vi "Passmark_Setting_Save.vi"(7 "Table_Data 2":refnum<vi>, 8 "error in (no error)":errorcluster caption="错误输入（无错误）", 9 "GRR_Title_Setting_path":path=path "D:/Desktop/?????/Title_RecipeEVT3_GRR.csv", 10 "Title_Setting_path":path=path "D:/Desktop/?????/Title_RecipeEVT3.csv", 11 "Flow_Setting_path":path=path "D:/Desktop/?????/EOL_Passmark_Setting_RecipeEVT3.csv") -> (0 "error out":errorcluster caption="错误输出")   [LabVIEW 2017]
uses:
  <vilib>/Utility/file.llb/Read Delimited Spreadsheet (string).vi
  <vilib>/Utility/file.llb/Write Delimited Spreadsheet (string).vi
panel:
  out "GRR_Title_Setting_path 2":path
  out "Title_Setting_path 2":path
  out "Flow_Setting_path 2":path
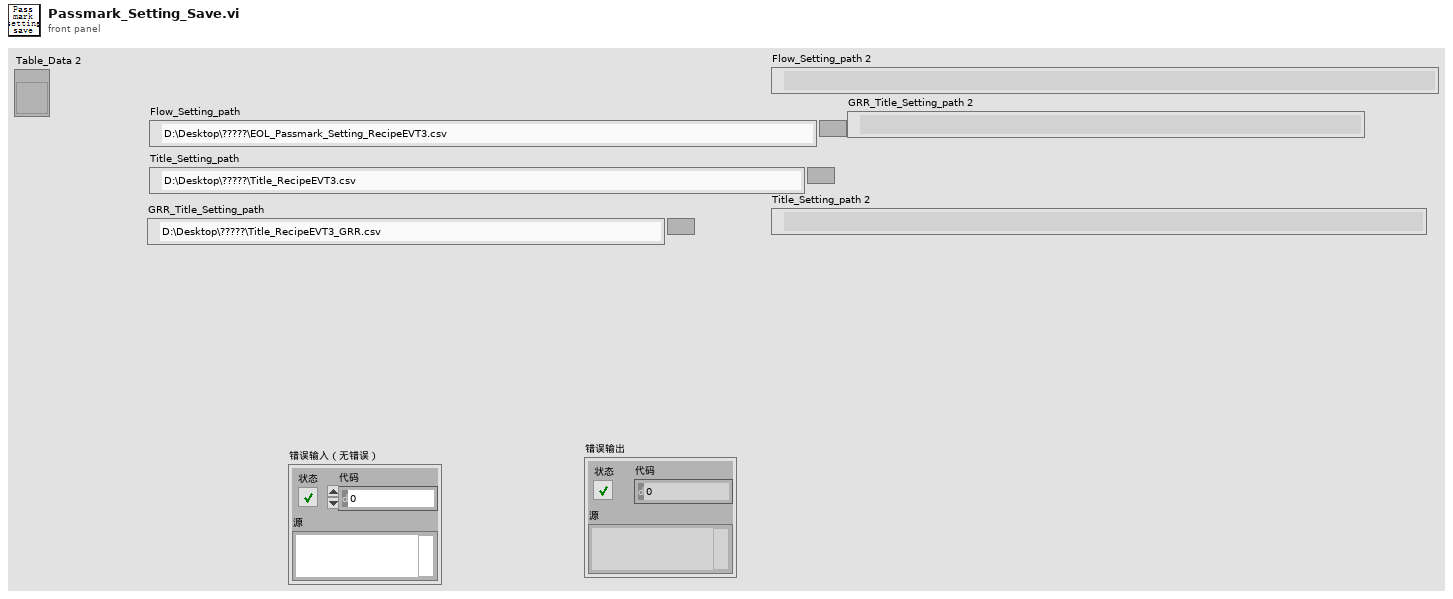
[diagram p1: front panel]
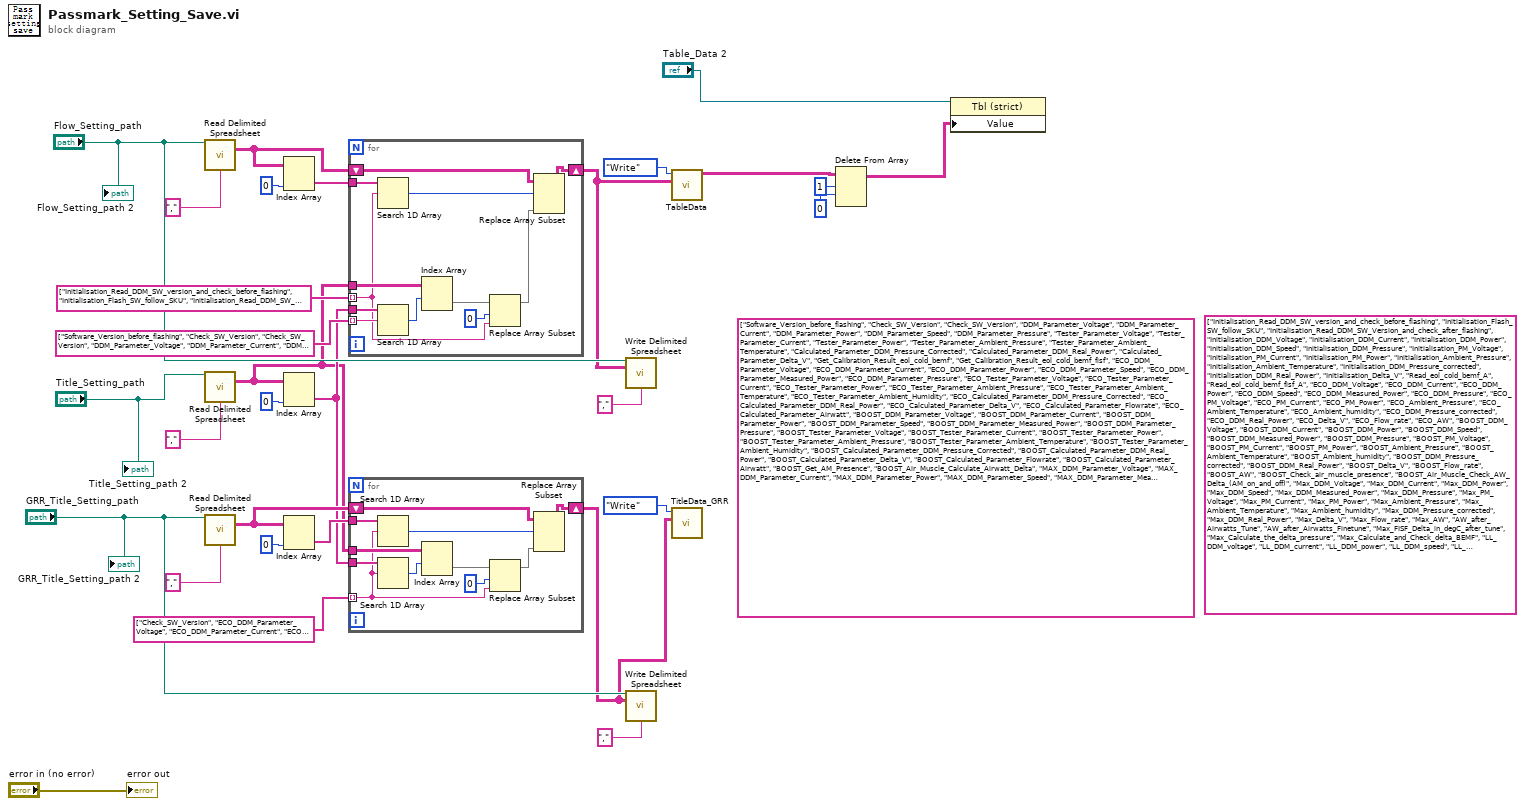
[diagram p0: block diagram]
diagram:
  (unwired) string[] ["Initialisation_Read_DDM_SW_version_and_check_before_flashing", "Initialisation_Flash_SW_follow_SKU", "Initialisation_Read_DDM_SW_Version_and_check_after_flashing", "Initialisation_DDM_Voltage", "Initialisation_DDM_Current", "Initialisation_DDM_Power", "Initialisation_DDM_Speed", "Initialisation_DDM_Pressure", "Initialisation_PM_Voltage", "Initialisation_PM_Current", "Initialisation_PM_Power", "Initialisation_Ambient_Pressure", "Initialisation_Ambient_Temperature", "Initialisation_DDM_Pressure_corrected", "Initialisation_DDM_Real_Power", "Initialisation_Delta_V", "Read_eol_cold_bemf_A", "Read_eol_cold_bemf_fisf_A", "ECO_DDM_Voltage", "ECO_DDM_Current", "ECO_DDM_Power", "ECO_DDM_Speed", "ECO_DDM_Measured_Power", "ECO_DDM_Pressure", "ECO_PM_Voltage", "ECO_PM_Current", "ECO_PM_Power", "ECO_Ambient_Pressure", "ECO_Ambient_Temperature", "ECO_Ambient_humidity", "ECO_DDM_Pressure_corrected", "ECO_DDM_Real_Power", "ECO_Delta_V", "ECO_Flow_rate", "ECO_AW", "BOOST_DDM_Voltage", "BOOST_DDM_Current", "BOOST_DDM_Power", "BOOST_DDM_Speed", "BOOST_DDM_Measured_Power", "BOOST_DDM_Pressure", "BOOST_PM_Voltage", "BOOST_PM_Current", "BOOST_PM_Power", "BOOST_Ambient_Pressure", "BOOST_Ambient_Temperature", "BOOST_Ambient_humidity", "BOOST_DDM_Pressure_corrected", "BOOST_DDM_Real_Power", "BOOST_Delta_V", "BOOST_Flow_rate", "BOOST_AW", "BOOST_Check_air_muscle_presence", "BOOST_Air_Muscle_Check_AW_Delta_(AM_on_and_off)", "Max_DDM_Voltage", "Max_DDM_Current", "Max_DDM_Power", "Max_DDM_Speed", "Max_DDM_Measured_Power", "Max_DDM_Pressure", "Max_PM_Voltage", "Max_PM_Current", "Max_PM_Power", "Max_Ambient_Pressure", "Max_Ambient_Temperature", "Max_Ambient_humidity", "Max_DDM_Pressure_corrected", "Max_DDM_Real_Power", "Max_Delta_V", "Max_Flow_rate", "Max_AW", "AW_after_Airwatts_Tune", "AW_after_Airwatts_Finetune", "Max_FISF_Delta_in_degC_after_tune", "Max_Calculate_the_delta_pressure", "Max_Calculate_and_Check_delta_BEMF", "LL_DDM_voltage", "LL_DDM_current", "LL_DDM_power", "LL_DDM_speed", "LL_DDM_measured_power", "LL_DDM_pressure", "LL_Tester_Voltage", "LL_Tester_Current", "LL_Tester_Power", "LL_DDM_Real_Power", "Calibrate_task_detect-LL(A)", "HL_DDM_voltage", "HL_DDM_current", "HL_DDM_power", "HL_DDM_speed", "HL_DDM_measured_power", "HL_DDM_pressure", "HL_Tester_Voltage", "HL_Tester_Current", "HL_Tester_Power", "HL_DDM_Real_Power", "Calibrate_task_detect-HL(B)", "LH_DDM_voltage", "LH_DDM_current", "LH_DDM_power", "LH_DDM_speed", "LH_DDM_measured_power", "LH_DDM_pressure", "LH_Tester_Voltage", "LH_Tester_Current", "LH_Tester_Power", "LH_DDM_Real_Power", "Calibrate_task_detect-LH(C)", "HH_DDM_voltage", "HH_DDM_current", "HH_DDM_power", "HH_DDM_speed", "HH_DDM_measured_power", "HH_DDM_pressure", "HH_Tester_Voltage", "HH_Tester_Current", "HH_Tester_Power", "HH_DDM_Real_Power", "Calibrate_task_detect-HH(D)", "Inlet_Blockage_Calibration_DDM_voltage", "Inlet_Blockage_Calibration_DDM_current", "Inlet_Blockage_Calibration_DDM_power", "Inlet_Blockage_Calibration_DDM_speed", "Inlet_Blockage_Calibration_DDM_measured_power", "Inlet_Blockage_Calibration_pressure", "Inlet_Blockage_Calibration_Tester_Voltage", "Inlet_Blockage_Calibration_Tester_Current", "Inlet_Blockage_Calibration_Tester_Power", "Inlet_Blockage_Calibration_DDM_Real_Power", "HH_Get_inlet_blockage_calibration(E)"] ("子数组 3")
  (unwired) string[] ["Software_Version_before_flashing", "Check_SW_Version", "Check_SW_Version", "DDM_Parameter_Voltage", "DDM_Parameter_Current", "DDM_Parameter_Power", "DDM_Parameter_Speed", "DDM_Parameter_Pressure", "Tester_Parameter_Voltage", "Tester_Parameter_Current", "Tester_Parameter_Power", "Tester_Parameter_Ambient_Pressure", "Tester_Parameter_Ambient_Temperature", "Calculated_Parameter_DDM_Pressure_Corrected", "Calculated_Parameter_DDM_Real_Power", "Calculated_Parameter_Delta_V", "Get_Calibration_Result_eol_cold_bemf", "Get_Calibration_Result_eol_cold_bemf_fisf", "ECO_DDM_Parameter_Voltage", "ECO_DDM_Parameter_Current", "ECO_DDM_Parameter_Power", "ECO_DDM_Parameter_Speed", "ECO_DDM_Parameter_Measured_Power", "ECO_DDM_Parameter_Pressure", "ECO_Tester_Parameter_Voltage", "ECO_Tester_Parameter_Current", "ECO_Tester_Parameter_Power", "ECO_Tester_Parameter_Ambient_Pressure", "ECO_Tester_Parameter_Ambient_Temperature", "ECO_Tester_Parameter_Ambient_Humidity", "ECO_Calculated_Parameter_DDM_Pressure_Corrected", "ECO_Calculated_Parameter_DDM_Real_Power", "ECO_Calculated_Parameter_Delta_V", "ECO_Calculated_Parameter_Flowrate", "ECO_Calculated_Parameter_Airwatt", "BOOST_DDM_Parameter_Voltage", "BOOST_DDM_Parameter_Current", "BOOST_DDM_Parameter_Power", "BOOST_DDM_Parameter_Speed", "BOOST_DDM_Parameter_Measured_Power", "BOOST_DDM_Parameter_Pressure", "BOOST_Tester_Parameter_Voltage", "BOOST_Tester_Parameter_Current", "BOOST_Tester_Parameter_Power", "BOOST_Tester_Parameter_Ambient_Pressure", "BOOST_Tester_Parameter_Ambient_Temperature", "BOOST_Tester_Parameter_Ambient_Humidity", "BOOST_Calculated_Parameter_DDM_Pressure_Corrected", "BOOST_Calculated_Parameter_DDM_Real_Power", "BOOST_Calculated_Parameter_Delta_V", "BOOST_Calculated_Parameter_Flowrate", "BOOST_Calculated_Parameter_Airwatt", "BOOST_Get_AM_Presence", "BOOST_Air_Muscle_Calculate_Airwatt_Delta", "MAX_DDM_Parameter_Voltage", "MAX_DDM_Parameter_Current", "MAX_DDM_Parameter_Power", "MAX_DDM_Parameter_Speed", "MAX_DDM_Parameter_Measured_Power", "MAX_DDM_Parameter_Pressure", "MAX_Tester_Parameter_Voltage", "MAX_Tester_Parameter_Current", "MAX_Tester_Parameter_Power", "MAX_Tester_Parameter_Ambient_Pressure", "MAX_Tester_Parameter_Ambient_Temperature", "MAX_Tester_Parameter_Ambient_Humidity", "MAX_Calculated_Parameter_DDM_Pressure_Corrected", "MAX_Calculated_Parameter_DDM_Real_Power", "MAX_Calculated_Parameter_Delta_V", "MAX_Calculated_Parameter_Flowrate", "MAX_Calculated_Parameter_Airwatt", "MAX_tune_Calculated_Parameter_Airwatt", "MAX_finetune_Calculated_Parameter_Airwatt", "Delta_Tmag_FISF", "Calculate_delta_Pressure", "Calculate_Check_Delta_BEMF", "LL_DDM_Parameter_Voltage", "LL_DDM_Parameter_Current", "LL_DDM_Parameter_Power", "LL_DDM_Parameter_Speed", "LL_DDM_Parameter_Measured_Power", "LL_DDM_Parameter_Pressure", "LL_Tester_Parameter_Voltage", "LL_Tester_Parameter_Current", "LL_Tester_Parameter_Power", "LL_DDM_Real_Power", "LL_Calibrate_Task_Detect_LL", "HL_DDM_Parameter_Voltage", "HL_DDM_Parameter_Current", "HL_DDM_Parameter_Power", "HL_DDM_Parameter_Speed", "HL_DDM_Parameter_Measured_Power", "HL_DDM_Parameter_Pressure", "HL_Tester_Parameter_Voltage", "HL_Tester_Parameter_Current", "HL_Tester_Parameter_Power", "HL_DDM_Real_Power", "HL_Calibrate_Task_Detect_HL", "LH_DDM_Parameter_Voltage", "LH_DDM_Parameter_Current", "LH_DDM_Parameter_Power", "LH_DDM_Parameter_Speed", "LH_DDM_Parameter_Measured_Power", "LH_DDM_Parameter_Pressure", "LH_Tester_Parameter_Voltage", "LH_Tester_Parameter_Current", "LH_Tester_Parameter_Power", "LH_DDM_Real_Power", "LH_Calibrate_Task_Detect_LH", "HH_DDM_Parameter_Voltage", "HH_DDM_Parameter_Current", "HH_DDM_Parameter_Power", "HH_DDM_Parameter_Speed", "HH_DDM_Parameter_Measured_Power", "HH_DDM_Parameter_Pressure", "HH_Tester_Parameter_Voltage", "HH_Tester_Parameter_Current", "HH_Tester_Parameter_Power", "HH_DDM_Real_Power", "HH_Calibrate_Task_Detect_HH", "Inlet_Blockage_Calibration_DDM_Parameter_Voltage", "Inlet_Blockage_Calibration_DDM_Parameter_Current", "Inlet_Blockage_Calibration_DDM_Parameter_Power", "Inlet_Blockage_Calibration_DDM_Parameter_Speed", "Inlet_Blockage_Calibration_DDM_Parameter_Measured_Power", "Inlet_Blockage_Calibration_DDM_Parameter_Pressure", "Inlet_Blockage_Calibration_Tester_Parameter_Voltage", "Inlet_Blockage_Calibration_Tester_Parameter_Current", "Inlet_Blockage_Calibration_Tester_Parameter_Power", "Inlet_Blockage_Calibration_DDM_Real_Power", "Calibration_Inlet_Blockage"] ("子数组 3")
  n1 = call-poly <vilib>:"Read Delimited Spreadsheet.vi"("file path (dialog if empty)"="Flow_Setting_path", "delimiter (\\t)"="," ("delimiter (\\t)")) -> ("all rows"=w25:string[][])  [unwired: 8 in, 5 out]
  n2 = call-poly <vilib>:"Read Delimited Spreadsheet.vi"("file path (dialog if empty)"="Title_Setting_path", "delimiter (\\t)"="," ("delimiter (\\t)")) -> ("all rows"=w11:string[][])  [unwired: 8 in, 5 out]
  n3 = call-poly <vilib>:"Read Delimited Spreadsheet.vi"("file path (dialog if empty)"="GRR_Title_Setting_path", "delimiter (\\t)"="," ("delimiter (\\t)")) -> ("all rows"=w18:string[][])  [unwired: 8 in, 5 out]
  n4 = Index Array(array=w25, index (col)=0 ("禁用的索引 (列)")) -> (element=w22:string[])  [unwired: 1 in]
  n5 = Index Array(array=w11, index (col)=0 ("禁用的索引 (列)")) -> (element=w12:string[])  [unwired: 1 in]
  n6 = Index Array(array=w18, index (col)=0 ("禁用的索引 (列)")) -> (element=w17:string[])  [unwired: 1 in]
  n7 = for {
    tunnel: string[] ["Initialisation_Read_DDM_SW_version_and_check_before_flashing", "Initialisation_Flash_SW_follow_SKU", "Initialisation_Read_DDM_SW_Version_and_check_after_flashing", "Initialisation_DDM_Voltage", "Initialisation_DDM_Current", "Initialisation_DDM_Power", "Initialisation_DDM_Speed", "Initialisation_DDM_Pressure", "Initialisation_PM_Voltage", "Initialisation_PM_Current", "Initialisation_PM_Power", "Initialisation_Ambient_Pressure", "Initialisation_Ambient_Temperature", "Initialisation_DDM_Pressure_corrected", "Initialisation_DDM_Real_Power", "Initialisation_Delta_V", "Read_eol_cold_bemf_A", "Read_eol_cold_bemf_fisf_A", "ECO_DDM_Voltage", "ECO_DDM_Current", "ECO_DDM_Power", "ECO_DDM_Speed", "ECO_DDM_Measured_Power", "ECO_DDM_Pressure", "ECO_PM_Voltage", "ECO_PM_Current", "ECO_PM_Power", "ECO_Ambient_Pressure", "ECO_Ambient_Temperature", "ECO_Ambient_humidity", "ECO_DDM_Pressure_corrected", "ECO_DDM_Real_Power", "ECO_Delta_V", "ECO_Flow_rate", "ECO_AW", "BOOST_DDM_Voltage", "BOOST_DDM_Current", "BOOST_DDM_Power", "BOOST_DDM_Speed", "BOOST_DDM_Measured_Power", "BOOST_DDM_Pressure", "BOOST_PM_Voltage", "BOOST_PM_Current", "BOOST_PM_Power", "BOOST_Ambient_Pressure", "BOOST_Ambient_Temperature", "BOOST_Ambient_humidity", "BOOST_DDM_Pressure_corrected", "BOOST_DDM_Real_Power", "BOOST_Delta_V", "BOOST_Flow_rate", "BOOST_AW", "BOOST_Check_air_muscle_presence", "BOOST_Air_Muscle_Check_AW_Delta_(AM_on_and_off)", "Max_DDM_Voltage", "Max_DDM_Current", "Max_DDM_Power", "Max_DDM_Speed", "Max_DDM_Measured_Power", "Max_DDM_Pressure", "Max_PM_Voltage", "Max_PM_Current", "Max_PM_Power", "Max_Ambient_Pressure", "Max_Ambient_Temperature", "Max_Ambient_humidity", "Max_DDM_Pressure_corrected", "Max_DDM_Real_Power", "Max_Delta_V", "Max_Flow_rate", "Max_AW", "AW_after_Airwatts_Tune", "AW_after_Airwatts_Finetune", "Max_FISF_Delta_in_degC_after_tune", "Max_Calculate_the_delta_pressure", "Max_Calculate_and_Check_delta_BEMF", "LL_DDM_voltage", "LL_DDM_current", "LL_DDM_power", "LL_DDM_speed", "LL_DDM_measured_power", "LL_DDM_pressure", "LL_Tester_Voltage", "LL_Tester_Current", "LL_Tester_Power", "LL_DDM_Real_Power", "Calibrate_task_detect-LL(A)", "HL_DDM_voltage", "HL_DDM_current", "HL_DDM_power", "HL_DDM_speed", "HL_DDM_measured_power", "HL_DDM_pressure", "HL_Tester_Voltage", "HL_Tester_Current", "HL_Tester_Power", "HL_DDM_Real_Power", "Calibrate_task_detect-HL(B)", "LH_DDM_voltage", "LH_DDM_current", "LH_DDM_power", "LH_DDM_speed", "LH_DDM_measured_power", "LH_DDM_pressure", "LH_Tester_Voltage", "LH_Tester_Current", "LH_Tester_Power", "LH_DDM_Real_Power", "Calibrate_task_detect-LH(C)", "HH_DDM_voltage", "HH_DDM_current", "HH_DDM_power", "HH_DDM_speed", "HH_DDM_measured_power", "HH_DDM_pressure", "HH_Tester_Voltage", "HH_Tester_Current", "HH_Tester_Power", "HH_DDM_Real_Power", "Calibrate_task_detect-HH(D)", "Inlet_Blockage_Calibration_DDM_voltage", "Inlet_Blockage_Calibration_DDM_current", "Inlet_Blockage_Calibration_DDM_power", "Inlet_Blockage_Calibration_DDM_speed", "Inlet_Blockage_Calibration_DDM_measured_power", "Inlet_Blockage_Calibration_pressure", "Inlet_Blockage_Calibration_Tester_Voltage", "Inlet_Blockage_Calibration_Tester_Current", "Inlet_Blockage_Calibration_Tester_Power", "Inlet_Blockage_Calibration_DDM_Real_Power", "HH_Get_inlet_blockage_calibration(E)"] ("子数组 3") -> [w33] mode=indexing
    tunnel: string[] ["Software_Version_before_flashing", "Check_SW_Version", "Check_SW_Version", "DDM_Parameter_Voltage", "DDM_Parameter_Current", "DDM_Parameter_Power", "DDM_Parameter_Speed", "DDM_Parameter_Pressure", "Tester_Parameter_Voltage", "Tester_Parameter_Current", "Tester_Parameter_Power", "Tester_Parameter_Ambient_Pressure", "Tester_Parameter_Ambient_Temperature", "Calculated_Parameter_DDM_Pressure_Corrected", "Calculated_Parameter_DDM_Real_Power", "Calculated_Parameter_Delta_V", "Get_Calibration_Result_eol_cold_bemf", "Get_Calibration_Result_eol_cold_bemf_fisf", "ECO_DDM_Parameter_Voltage", "ECO_DDM_Parameter_Current", "ECO_DDM_Parameter_Power", "ECO_DDM_Parameter_Speed", "ECO_DDM_Parameter_Measured_Power", "ECO_DDM_Parameter_Pressure", "ECO_Tester_Parameter_Voltage", "ECO_Tester_Parameter_Current", "ECO_Tester_Parameter_Power", "ECO_Tester_Parameter_Ambient_Pressure", "ECO_Tester_Parameter_Ambient_Temperature", "ECO_Tester_Parameter_Ambient_Humidity", "ECO_Calculated_Parameter_DDM_Pressure_Corrected", "ECO_Calculated_Parameter_DDM_Real_Power", "ECO_Calculated_Parameter_Delta_V", "ECO_Calculated_Parameter_Flowrate", "ECO_Calculated_Parameter_Airwatt", "BOOST_DDM_Parameter_Voltage", "BOOST_DDM_Parameter_Current", "BOOST_DDM_Parameter_Power", "BOOST_DDM_Parameter_Speed", "BOOST_DDM_Parameter_Measured_Power", "BOOST_DDM_Parameter_Pressure", "BOOST_Tester_Parameter_Voltage", "BOOST_Tester_Parameter_Current", "BOOST_Tester_Parameter_Power", "BOOST_Tester_Parameter_Ambient_Pressure", "BOOST_Tester_Parameter_Ambient_Temperature", "BOOST_Tester_Parameter_Ambient_Humidity", "BOOST_Calculated_Parameter_DDM_Pressure_Corrected", "BOOST_Calculated_Parameter_DDM_Real_Power", "BOOST_Calculated_Parameter_Delta_V", "BOOST_Calculated_Parameter_Flowrate", "BOOST_Calculated_Parameter_Airwatt", "BOOST_Get_AM_Presence", "BOOST_Air_Muscle_Calculate_Airwatt_Delta", "MAX_DDM_Parameter_Voltage", "MAX_DDM_Parameter_Current", "MAX_DDM_Parameter_Power", "MAX_DDM_Parameter_Speed", "MAX_DDM_Parameter_Measured_Power", "MAX_DDM_Parameter_Pressure", "MAX_Tester_Parameter_Voltage", "MAX_Tester_Parameter_Current", "MAX_Tester_Parameter_Power", "MAX_Tester_Parameter_Ambient_Pressure", "MAX_Tester_Parameter_Ambient_Temperature", "MAX_Tester_Parameter_Ambient_Humidity", "MAX_Calculated_Parameter_DDM_Pressure_Corrected", "MAX_Calculated_Parameter_DDM_Real_Power", "MAX_Calculated_Parameter_Delta_V", "MAX_Calculated_Parameter_Flowrate", "MAX_Calculated_Parameter_Airwatt", "MAX_tune_Calculated_Parameter_Airwatt", "MAX_finetune_Calculated_Parameter_Airwatt", "Delta_Tmag_FISF", "Calculate_delta_Pressure", "Calculate_Check_Delta_BEMF", "LL_DDM_Parameter_Voltage", "LL_DDM_Parameter_Current", "LL_DDM_Parameter_Power", "LL_DDM_Parameter_Speed", "LL_DDM_Parameter_Measured_Power", "LL_DDM_Parameter_Pressure", "LL_Tester_Parameter_Voltage", "LL_Tester_Parameter_Current", "LL_Tester_Parameter_Power", "LL_DDM_Real_Power", "LL_Calibrate_Task_Detect_LL", "HL_DDM_Parameter_Voltage", "HL_DDM_Parameter_Current", "HL_DDM_Parameter_Power", "HL_DDM_Parameter_Speed", "HL_DDM_Parameter_Measured_Power", "HL_DDM_Parameter_Pressure", "HL_Tester_Parameter_Voltage", "HL_Tester_Parameter_Current", "HL_Tester_Parameter_Power", "HL_DDM_Real_Power", "HL_Calibrate_Task_Detect_HL", "LH_DDM_Parameter_Voltage", "LH_DDM_Parameter_Current", "LH_DDM_Parameter_Power", "LH_DDM_Parameter_Speed", "LH_DDM_Parameter_Measured_Power", "LH_DDM_Parameter_Pressure", "LH_Tester_Parameter_Voltage", "LH_Tester_Parameter_Current", "LH_Tester_Parameter_Power", "LH_DDM_Real_Power", "LH_Calibrate_Task_Detect_LH", "HH_DDM_Parameter_Voltage", "HH_DDM_Parameter_Current", "HH_DDM_Parameter_Power", "HH_DDM_Parameter_Speed", "HH_DDM_Parameter_Measured_Power", "HH_DDM_Parameter_Pressure", "HH_Tester_Parameter_Voltage", "HH_Tester_Parameter_Current", "HH_Tester_Parameter_Power", "HH_DDM_Real_Power", "HH_Calibrate_Task_Detect_HH", "Inlet_Blockage_Calibration_DDM_Parameter_Voltage", "Inlet_Blockage_Calibration_DDM_Parameter_Current", "Inlet_Blockage_Calibration_DDM_Parameter_Power", "Inlet_Blockage_Calibration_DDM_Parameter_Speed", "Inlet_Blockage_Calibration_DDM_Parameter_Measured_Power", "Inlet_Blockage_Calibration_DDM_Parameter_Pressure", "Inlet_Blockage_Calibration_Tester_Parameter_Voltage", "Inlet_Blockage_Calibration_Tester_Parameter_Current", "Inlet_Blockage_Calibration_Tester_Parameter_Power", "Inlet_Blockage_Calibration_DDM_Real_Power", "Calibration_Inlet_Blockage"] ("子数组 3") -> [w41] mode=indexing
    tunnel: w11 -> [w39]
    tunnel: w12 -> [w42]
    tunnel: w22 -> [w40]
    shift-right: [w37] -> w8
    shift-left: w25 -> [w36]
    n8 = Search 1D Array(1D array=w40, element=w33) -> (index of element=w35:i32)  [unwired: 1 in]
    n9 = Search 1D Array(1D array=w42, element=w41) -> (index of element=w38:i32)  [unwired: 1 in]
    n10 = Index Array(array=w39, index (row)=w38) -> (element=w34:string[])  [unwired: 1 in]
    n11 = Replace Array Subset(array=w34, new element=w33, index=0 ("索引")) -> (w31:string[])
    n12 = Replace Array Subset ("替换数组子集")(array=w36, new element=w31, index (row)=w35) -> (w37:string[][])  [unwired: 1 in]
  }
  n13 = for {
    tunnel: string[] ["Check_SW_Version", "ECO_DDM_Parameter_Voltage", "ECO_DDM_Parameter_Current", "ECO_DDM_Parameter_Power", "ECO_DDM_Parameter_Measured_Power", "ECO_DDM_Parameter_Speed", "ECO_DDM_Parameter_Pressure", "ECO_Tester_Parameter_Voltage", "ECO_Tester_Parameter_Current", "ECO_Tester_Parameter_Power", "ECO_Tester_Parameter_Ambient_Pressure", "ECO_Tester_Parameter_Ambient_Temperature", "ECO_Tester_Parameter_Ambient_Humidity", "ECO_Calculated_Parameter_DDM_Pressure_Corrected", "ECO_Calculated_Parameter_DDM_Real_Power", "ECO_Calculated_Parameter_Delta_V", "ECO_Calculated_Parameter_Flowrate", "ECO_Calculated_Parameter_Airwatt", "BOOST_DDM_Parameter_Voltage", "BOOST_DDM_Parameter_Current", "BOOST_DDM_Parameter_Power", "BOOST_DDM_Parameter_Measured_Power", "BOOST_DDM_Parameter_Speed", "BOOST_DDM_Parameter_Pressure", "BOOST_Tester_Parameter_Voltage", "BOOST_Tester_Parameter_Current", "BOOST_Tester_Parameter_Power", "BOOST_Tester_Parameter_Ambient_Pressure", "BOOST_Tester_Parameter_Ambient_Temperature", "BOOST_Tester_Parameter_Ambient_Humidity", "BOOST_Calculated_Parameter_DDM_Pressure_Corrected", "BOOST_Calculated_Parameter_DDM_Real_Power", "BOOST_Calculated_Parameter_Delta_V", "BOOST_Calculated_Parameter_Flowrate", "BOOST_Calculated_Parameter_Airwatt", "MAX_DDM_Parameter_Voltage", "MAX_DDM_Parameter_Current", "MAX_DDM_Parameter_Power", "MAX_DDM_Parameter_Measured_Power", "MAX_DDM_Parameter_Speed", "MAX_DDM_Parameter_Pressure", "MAX_Tester_Parameter_Voltage", "MAX_Tester_Parameter_Current", "MAX_Tester_Parameter_Power", "MAX_Tester_Parameter_Ambient_Pressure", "MAX_Tester_Parameter_Ambient_Temperature", "MAX_Tester_Parameter_Ambient_Humidity", "MAX_Calculated_Parameter_DDM_Pressure_Corrected", "MAX_Calculated_Parameter_DDM_Real_Power", "MAX_Calculated_Parameter_Delta_V", "MAX_Calculated_Parameter_Flowrate", "MAX_Calculated_Parameter_Airwatt"] ("子数组") -> [w43] mode=indexing
    tunnel: w11 -> [w52]
    tunnel: w12 -> [w53]
    tunnel: w17 -> [w45]
    shift-right: [w50] -> w6
    shift-left: w18 -> [w44]
    n14 = Search 1D Array(1D array=w45, element=w43) -> (index of element=w49:i32)  [unwired: 1 in]
    n15 = Search 1D Array(1D array=w53, element=w43) -> (index of element=w51:i32)  [unwired: 1 in]
    n16 = Index Array(array=w52, index (row)=w51) -> (element=w48:string[])  [unwired: 1 in]
    n17 = Replace Array Subset(array=w48, new element=w43, index=0 ("索引")) -> (w46:string[])
    n18 = Replace Array Subset ("替换数组子集")(array=w44, new element=w46, index (row)=w49) -> (w50:string[][])  [unwired: 1 in]
  }
  n19 = call-poly <vilib>:"Write Delimited Spreadsheet.vi"("file path (dialog if empty)"="Flow_Setting_path", "2D data"=w8, "delimiter (\\t)"="," ("delimiter (\\t)")) -> ()  [unwired: 11 in, 2 out]
  n20 = call-poly <vilib>:"Write Delimited Spreadsheet.vi"("file path (dialog if empty)"="GRR_Title_Setting_path", "2D data"=w6, "delimiter (\\t)"="," ("delimiter (\\t)")) -> ()  [unwired: 11 in, 2 out]
  n21 = call "TableData.vi"("Tabledata in"=w8, "Step"=enum16{"Initial", "Write", "Read"}."Write") -> ("Tabledata Out"=w3:string[][])  [unwired: 8 in, 1 out]
  n22 = call "TitleData_GRR.vi"("Tabledata in"=w6, "Step"=enum16{"Initial", "Write", "Read"}."Write") -> ()  [unwired: 8 in, 2 out]
  n23 = Delete From Array(array=w3, length=1 ("长度"), index (row)=0 ("索引 (行)")) -> (array with subset deleted=w1:string[][])  [unwired: 1 in, 1 out]
  n24 = property class="Tbl (strict)"(reference="Table_Data 2", "Value"=w1) -> ()  [unwired: 1 in, 2 out]
  "error out" <- "error in (no error)"
  "Flow_Setting_path 2" <- "Flow_Setting_path"
  "Title_Setting_path 2" <- "Title_Setting_path"
  "GRR_Title_Setting_path 2" <- "GRR_Title_Setting_path"
